vi "PS Settings Dialog.vi"(8 "error in":errorcluster, 9 "Model":string, 11 "Settings in":T1 {"Voltage Limit" scale=0.0..155.0 scale format="%.3g"; "Hardware Configuration"."Baud Rate" items=["<0>"=0, "4800"=4800, "9600"=9600, "19200"=19200, "38400"=38400, "57600"=57600, "115200"=115200]}) -> (0 "error out":errorcluster, 1 "Cancelled?":bool, 2 "UI Refresh Needed?":bool, 3 "Settings out":T1 {"Voltage Limit" scale=0.0..155.0 scale format="%.3g"; "Hardware Configuration"."Baud Rate" items=["<0>"=0, "4800"=4800, "9600"=9600, "19200"=19200, "38400"=38400, "57600"=57600, "115200"=115200]})   [LabVIEW 2022 SP3, in "Settings.lvlib"]
doc: "Dialog for selecting user specified settings."
uses:
  Settings.lvlib
  Settings.ctl
  Acquisition/Hardware Configuration.ctl
  Logging/Logging Configuration.ctl
  <vilib>/Utility/miscctls.llb/LVMinMaxIncTypeDef.ctl
  Acquisition/Acquisition.lvlib
  Logging/Logging.lvlib
panel:
  in  "OVP Delay":dbl=0.001 min=0.001 max=0.6 step=0.001
  in  "Voltage Limit":cluster{"Numeric":dbl, "Numeric":dbl}(slide)={"Numeric"=150.0, "Numeric"=0.0} scale=0.0..80.0 scale format="%.3g"
  in  "OVP State":bool=TRUE
  in  "Current Limit":dbl=30.0 min=0.0 max=61.0 step=1.0 format="%.3g"
  in  "OVP Limit":dbl=155.0 min=0.0 max=85.0 step=1.0 format="%.3g"
  in  "Cancel":bool
  in  "OK Button":bool
  # "Non visible portion of dialog (needed for connector pane)."
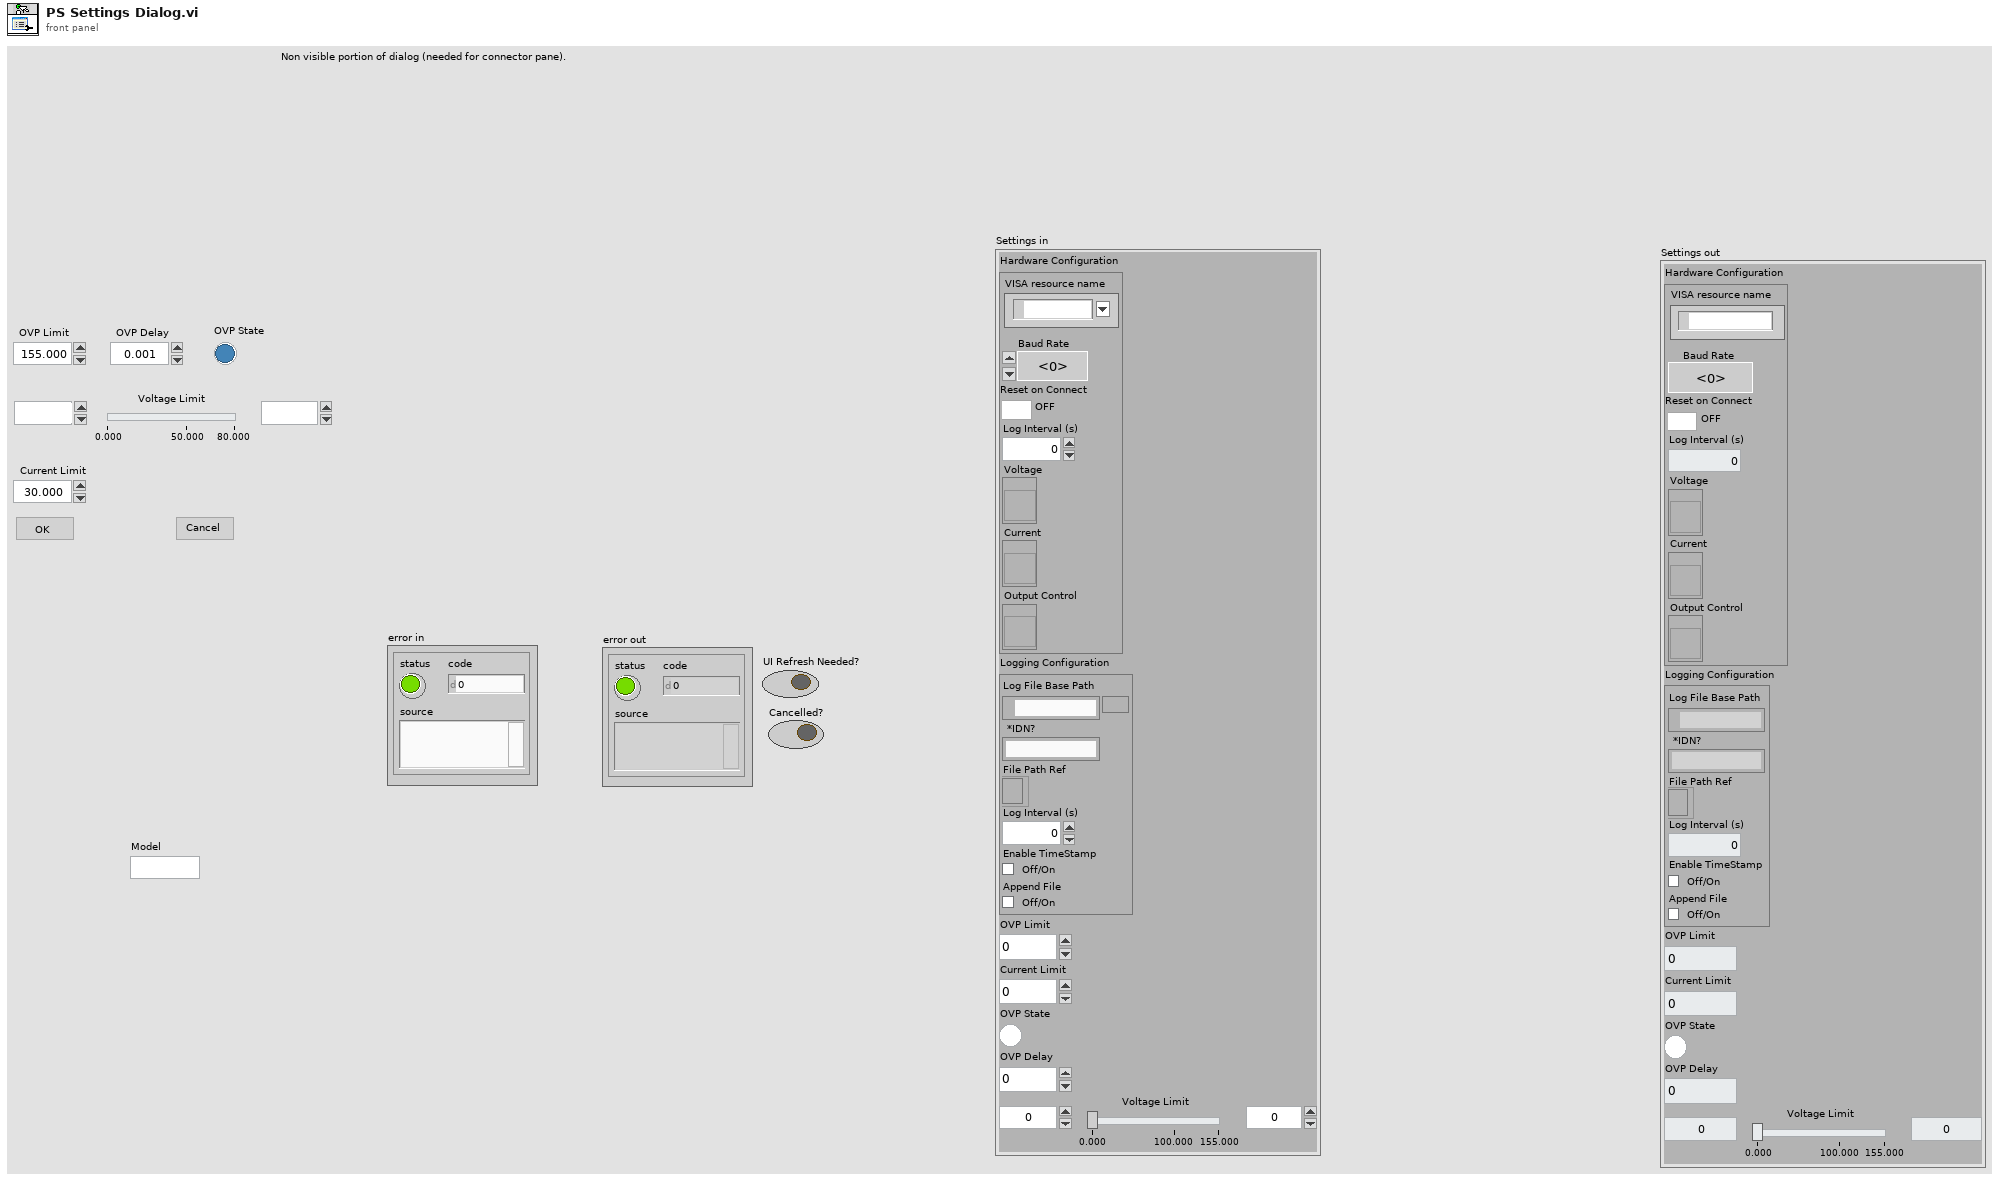
[diagram p1: front panel]
types:
  T1 = typedef "Settings.lvlib/Settings.ctl" = cluster{"Hardware Configuration":T2, "Logging Configuration":T3, "OVP Limit":dbl, "Current Limit":dbl, "OVP State":bool, "OVP Delay":dbl, "Voltage Limit":cluster{"Numeric":dbl, "Numeric":dbl}}
  T2 = typedef "Acquisition.lvlib/Hardware Configuration.ctl" = cluster{"VISA resource name":refnum<visa-resource-name>, "Baud Rate":u32, "Reset on Connect":bool, "Log Interval (s)":dbl, "Voltage":refnum<vi>, "Current":refnum<vi>, "Output Control":refnum<vi>}
  T3 = typedef "Logging.lvlib/Logging Configuration.ctl" = cluster{"Log File Base Path":path, "*IDN?":string, "File Path Ref":refnum<file>, "Log Interval (s)":dbl, "Enable TimeStamp":bool, "Append File":bool}
  T4 = typedef "LVMinMaxIncTypeDef.ctl" = cluster{"Minimum":dbl, "Maximum":dbl, "Increment":dbl}
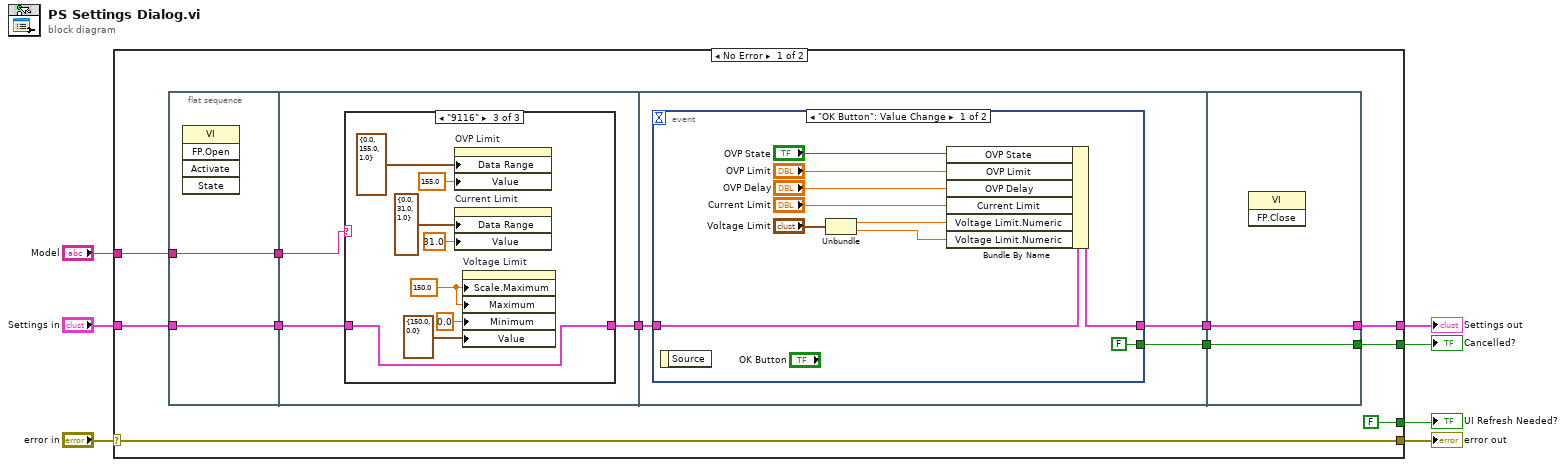
[diagram p0: block diagram]
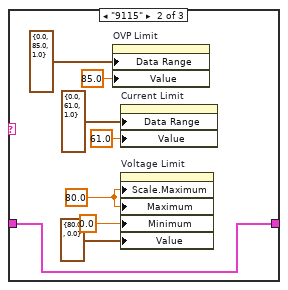
[diagram p3: hidden frame]
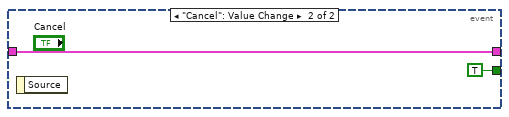
[diagram p4: hidden frame]
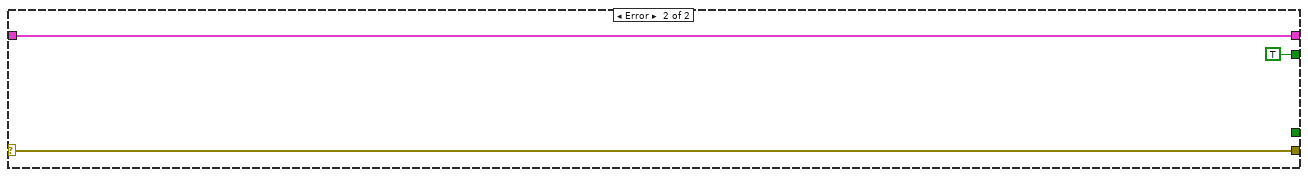
[diagram p5: hidden frame]
diagram:
  n1 = case shown="No Error" "error in" {
    selector: "error in" -> [w18 w60]
    tunnel: [w18 w60] -> w6
    tunnel: "Settings in" -> [w14 w59]
    tunnel: [w15 w59] -> w4
    tunnel: [FALSE ("UI Refresh Needed?") _] -> w3
    tunnel: [w16 TRUE ("UI Refresh Needed?")] -> w2
    tunnel: "Model" -> [w8 _]
    frame No Error {
      n2 = flat-sequence {
        tunnel: w14 -> [w20]
        tunnel: [w20] -> w11
        tunnel: [w19] -> w9
        tunnel: w8 -> [w19]
        tunnel: w11 -> [w22]
        tunnel: [w21] -> w10
        tunnel: w9 -> [w23]
        tunnel: w10 -> [w41]
        tunnel: [w43] -> w13
        tunnel: [w42] -> w12
        tunnel: [w56] -> w15
        tunnel: [w57] -> w16
        tunnel: w13 -> [w57]
        tunnel: w12 -> [w56]
        frame #0 {
          n3 = invoke class="VI" method="FP.Open"() -> ()  [unwired: 5 in, 5 out]
        }
        frame #1 {
          n4 = case shown="\"9116\"" w23 {
            tunnel: w22 -> [w24 w26 w33]
            tunnel: [w24 w26 w33] -> w21
            frame "False", Default {
            }
            frame "9115" {
              w30 = 80.0 ("Scale.Range:Maximum")
              n5 = property on="OVP Limit" class="DigNum (strict)"("Data Range"=T4 {"Minimum"=0.0, "Maximum"=85.0, "Increment"=1.0} ("Data Entry Limits"), "Value"=85.0 ("OVP Limit")) -> ()  [unwired: 2 in, 2 out]
              n6 = property on="Current Limit" class="DigNum (strict)"("Data Range"=T4 {"Minimum"=0.0, "Maximum"=61.0, "Increment"=1.0} ("Data Entry Limits"), "Value"=61.0 ("Current Limit")) -> ()  [unwired: 2 in, 2 out]
              n7 = property on="Voltage Limit" class="Slide (strict)"("Scale.Maximum"=w30, "Maximum"=w30, "Minimum"=0.0 ("Data Entry Limits:Minimum"), "Value"=cluster{"Numeric":dbl, "Numeric":dbl} {"Numeric"=80.0, "Numeric"=0.0} ("Voltage Limit")) -> ()  [unwired: 2 in, 2 out]
            }
            frame "9116" {
              w38 = 150.0 ("Scale.Range:Maximum")
              n8 = property on="OVP Limit" class="DigNum (strict)"("Data Range"=T4 {"Minimum"=0.0, "Maximum"=155.0, "Increment"=1.0} ("Data Entry Limits"), "Value"=155.0 ("OVP Limit")) -> ()  [unwired: 2 in, 2 out]
              n9 = property on="Current Limit" class="DigNum (strict)"("Data Range"=T4 {"Minimum"=0.0, "Maximum"=31.0, "Increment"=1.0} ("Data Entry Limits"), "Value"=31.0 ("Current Limit")) -> ()  [unwired: 2 in, 2 out]
              n10 = property on="Voltage Limit" class="Slide (strict)"("Scale.Maximum"=w38, "Maximum"=w38, "Minimum"=0.0 ("Data Entry Limits:Minimum"), "Value"=cluster{"Numeric":dbl, "Numeric":dbl} {"Numeric"=150.0, "Numeric"=0.0} ("Voltage Limit")) -> ()  [unwired: 2 in, 2 out]
            }
          }
        }
        frame #2 {
          n11 = event shown="[0] \"OK Button\": Value Change" {
            selector: _ -> [_ _]
            dyn-events: _ -> [_ _]
            timeout: _ -> [_ _]
            tunnel: [w51 w55] -> w42
            tunnel: w41 -> [w52 w55]
            tunnel: [FALSE ("UI Refresh Needed?") TRUE ("UI Refresh Needed?")] -> w43
            event "OK Button": Value Change {
              n12 = event-data() -> ()  [unwired: 1 in, 1 out]
              n13 = Unbundle("Voltage Limit") -> ("Numeric"=w49:dbl, "Numeric"=w48:dbl)
              n14 = Bundle By Name(cluster=w52, "OVP State"="OVP State", "OVP Limit"="OVP Limit", "OVP Delay"="OVP Delay", "Current Limit"="Current Limit", "Voltage Limit.Numeric"=w49, "Voltage Limit.Numeric"=w48) -> (w51:T1)
            }
            event "Cancel": Value Change {
              n15 = event-data() -> ()  [unwired: 1 in, 1 out]
            }
          }
        }
        frame #3 {
          n16 = invoke class="VI" method="FP.Close"() -> ()  [unwired: 3 in, 3 out]
        }
      }
    }
    frame Error {
    }
  }
  "UI Refresh Needed?" <- w3
  "error out" <- w6
  "Settings out" <- w4
  "Cancelled?" <- w2
